vi "peg-in-hole 2015-03-12 Test.vi"() -> ()   [LabVIEW 2013]
uses:
  ROS/Code/SubVIs/BaxterSide.ctl
  Arm Globals.vi
  ROS/Code/Console/Servers/ServerSubs/(nist) Arm Globals.vi
panel:
  in  "Load Pick Pose":bool
  out "Pick Hole":T1={"X"=602.0, "Y"=-377.0, "Z"=10.0, "O"=0.0, "A"=0.0, "T"=0.0}
  in  "Pick Pose":dbl[](array[numeric])=[47.63671869556711, -52.91015618954133, -0.7470703116463477, 100.65673816623291, 0.6372070305218848, 42.143554639343975, 3.186035152609424]
  out "Loops Remaining":i32=1
  out "Peg":i32=1
  out "Times":dbl[](array[numeric])
  out "Status":string="Test.4"
  in  "Stop":bool
  out "error out":errorcluster
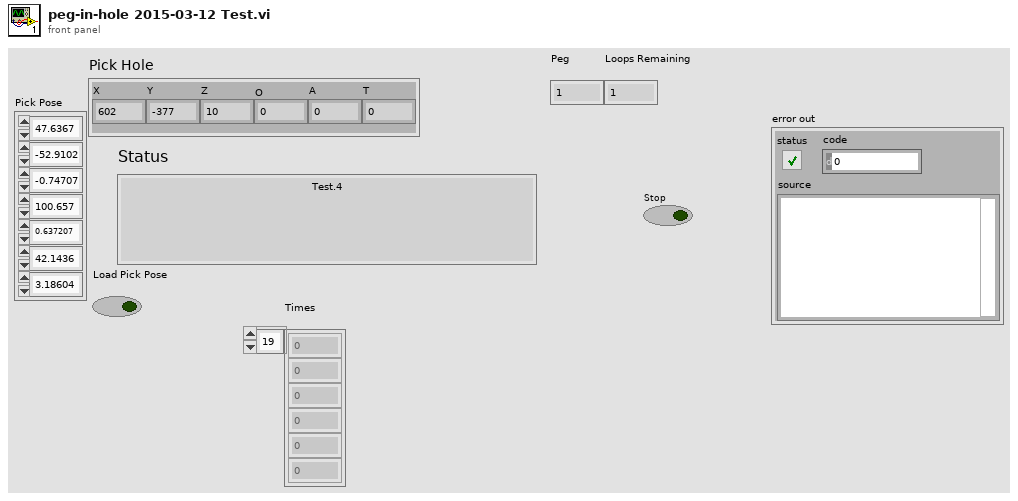
[diagram p1: front panel]
types:
  T1 = cluster{"X":dbl, "Y":dbl, "Z":dbl, "O":dbl, "A":dbl, "T":dbl}
  T2 = typedef "BaxterSide.ctl" = enum16{"left", "right"}
  T3 = cluster{"X":dbl, "Y":dbl, "Z":dbl, "O":dbl, "A":dbl, "T":dbl}[]
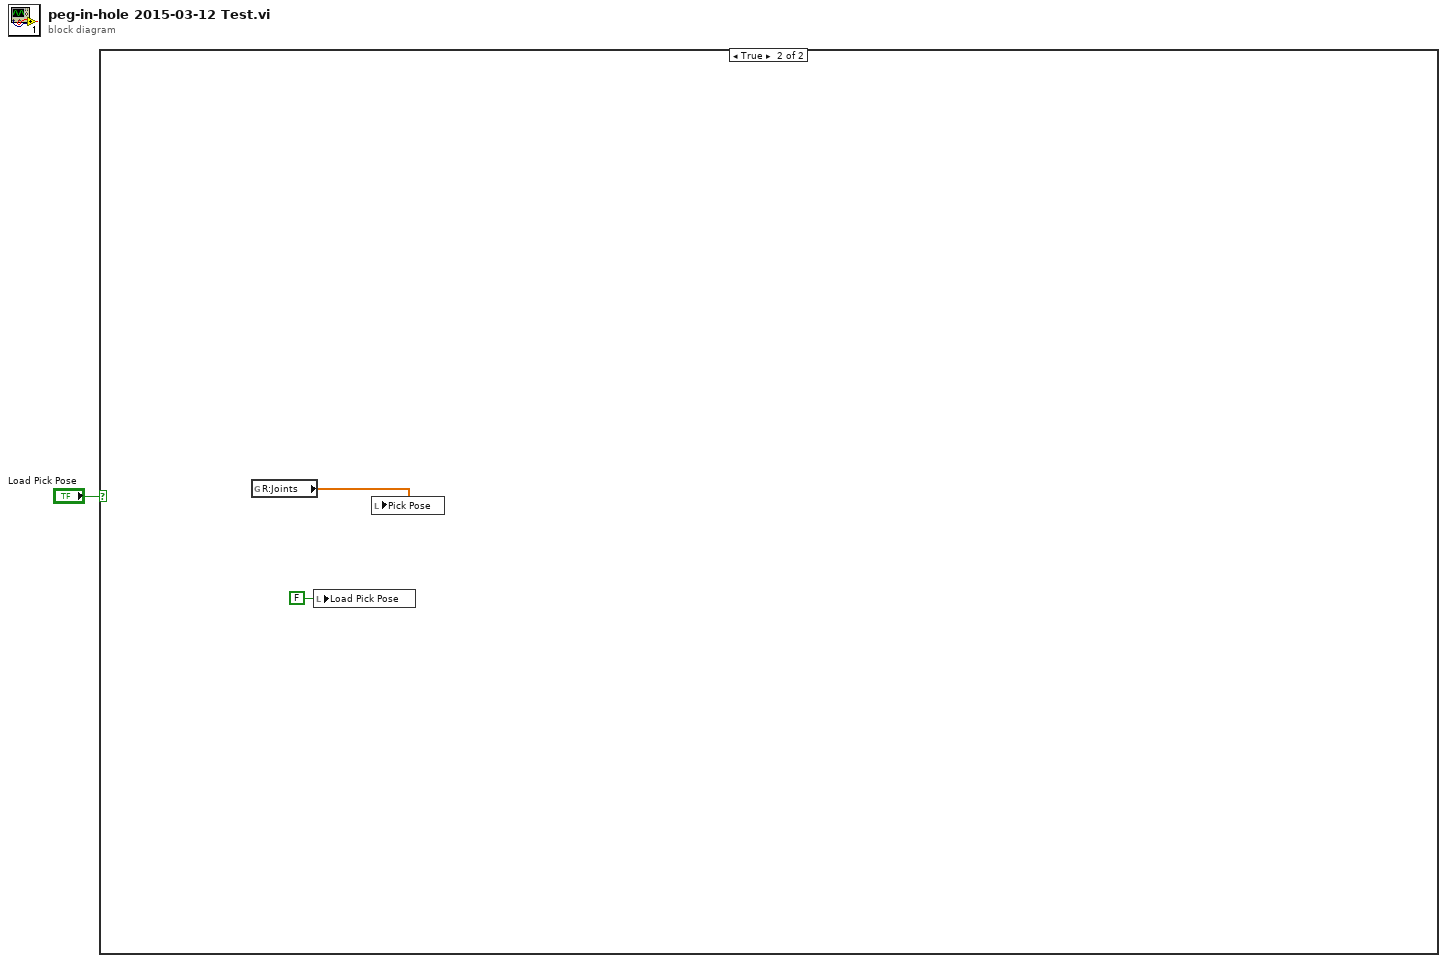
[diagram p0: block diagram]
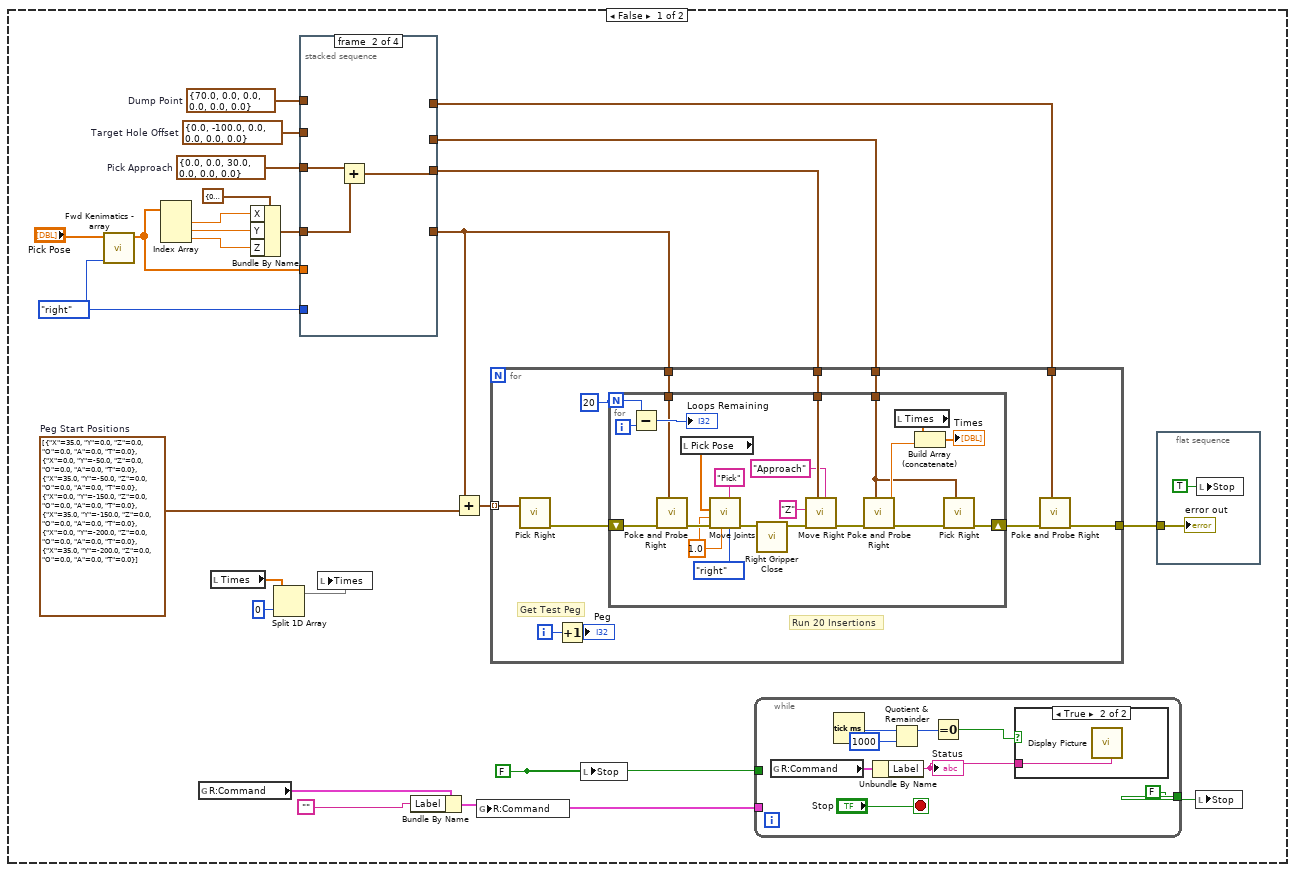
[diagram p2: hidden frame]
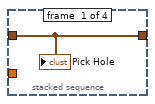
[diagram p3: hidden frame]
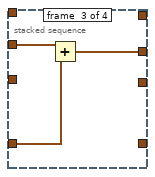
[diagram p4: hidden frame]
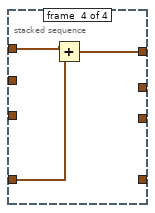
[diagram p5: hidden frame]
diagram:
  n1 = case shown="True" "Load Pick Pose" {
    frame False {
      w3 = T1 {"X"=0.0, "Y"=0.0, "Z"=30.0, "O"=0.0, "A"=0.0, "T"=0.0}  # Pick Approach
      w9 = T1 {"X"=70.0, "Y"=0.0, "Z"=0.0, "O"=0.0, "A"=0.0, "T"=0.0}  # Dump Point
      w10 = T1 {"X"=0.0, "Y"=-100.0, "Z"=0.0, "O"=0.0, "A"=0.0, "T"=0.0}  # Target Hole Offset
      w6 = BaxterSide."right" ("Side")
      w17 = T3 [{"X"=35.0, "Y"=0.0, "Z"=0.0, "O"=0.0, "A"=0.0, "T"=0.0}, {"X"=0.0, "Y"=-50.0, "Z"=0.0, "O"=0.0, "A"=0.0, "T"=0.0}, {"X"=35.0, "Y"=-50.0, "Z"=0.0, "O"=0.0, "A"=0.0, "T"=0.0}, {"X"=0.0, "Y"=-150.0, "Z"=0.0, "O"=0.0, "A"=0.0, "T"=0.0}, {"X"=35.0, "Y"=-150.0, "Z"=0.0, "O"=0.0, "A"=0.0, "T"=0.0}, {"X"=0.0, "Y"=-200.0, "Z"=0.0, "O"=0.0, "A"=0.0, "T"=0.0}, {"X"=35.0, "Y"=-200.0, "Z"=0.0, "O"=0.0, "A"=0.0, "T"=0.0}]  # Peg Start Positions
      w23 = FALSE ("Stop")
      n2 = call "Fwd Kenimatics - array.vi"("Side"=w6, "Joints"="Pick Pose") -> ("Position"=w7:dbl[])  [unwired: 8 in, 1 out]
      n3 = Index Array(array=w7) -> (element #1=w14:dbl, element #2=w13:dbl, element #3=w12:dbl)  [unwired: 3 in]
      n4 = global read "Arm Globals.vi" "R:Command"() -> (w27:cluster{"Label":string, "Angles":dbl[]})
      n5 = local read "Times"() -> (w21:dbl[])
      n6 = Bundle By Name(cluster=T1 {"X"=0.0, "Y"=0.0, "Z"=0.0, "O"=0.0, "A"=0.0, "T"=0.0} ("Pick Hole"), "X"=w14, "Y"=w13, "Z"=w12) -> (w11:T1)
      n7 = Split 1D Array(array=w21, index=0) -> (first subarray=w19:dbl[])  [unwired: 1 out]
      n8 = stacked-sequence {
        tunnel: w11 -> [w28 w30 w33 w36]
        tunnel: [w28 _ _ _] -> w5
        tunnel: w10 -> [_ _ w34 _]
        tunnel: [_ _ w32 _] -> w4
        tunnel: w9 -> [_ _ _ w37]
        tunnel: [_ _ _ w35] -> w8
        tunnel: w7 -> [_ _ _ _]
        tunnel: w6 -> [_ _ _ _]
        tunnel: w3 -> [_ w31 _ _]
        tunnel: [_ w29 _ _] -> w2
        frame #0 {
          "Pick Hole" <- w28
        }
        frame #1 {
          n9 = Add(x=w31, y=w30) -> (x+y=w29:T1)
        }
        frame #2 {
          n10 = Add(x=w34, y=w33) -> (x+y=w32:T1)
        }
        frame #3 {
          n11 = Add(x=w37, y=w36) -> (x+y=w35:T1)
        }
      }
      n12 = local write "Times"(w19) -> ()
      n13 = Bundle By Name(cluster=w27, "Label"="") -> (w25:cluster{"Label":string, "Angles":dbl[]})
      n14 = Add(x=w5, y=w17) -> (x+y=w18:T3)
      n15 = global write "Arm Globals.vi" "R:Command"(w25) -> ()
      n16 = for {
        tunnel: [w43] -> w22
        tunnel: w18 -> [w44] mode=indexing
        tunnel: w8 -> [w45]
        tunnel: w5 -> [w41]
        tunnel: w4 -> [w40]
        tunnel: w2 -> [w38]
        i -> [w46]
        # "Run 20 Insertions"
        # "Get Test Peg"
        n17 = call "Pick Right.vi"("Pick"=w44) -> ("error out"=w42:errorcluster)  [unwired: 10 in]
        n18 = Increment(x=w46) -> (x+1=→"Peg":i32)
        n19 = for {
          N: 20 -> [w68]
          shift-right: [w61] -> w39
          shift-left: w42 -> [w59]
          tunnel: w41 -> [w63]
          tunnel: w40 -> [w60]
          tunnel: w38 -> [w51]
          i -> [w67]
          w55 = 1.0 ("Wait (s)")
          n20 = Subtract(x=w68, y=w67) -> (x-y=→"Loops Remaining":i32)
          n21 = call "Poke and Probe Right.vi"("Start"=w63, "error in"=w59) -> ("error out"=w58:errorcluster)  [unwired: 8 in, 1 out]
          n22 = local read "Pick Pose"() -> (w56:dbl[])
          n23 = call "Move Joints.vi"("Side"=BaxterSide."right", "Label"="Pick", "Wait (s)"=w55, "error in"=w58, "time"=w55, "Goal"=w56) -> ("error out"=w54:errorcluster)  [unwired: 4 in, 1 out]
          n24 = call "Right Gripper Close.vi"("error in"=w54) -> ("error out"=w53:errorcluster)  [unwired: 9 in, 1 out]
          n25 = call "Move Right.vi"("Label"="Approach", "Goal Axes"=w51, "error in"=w53, "Mask"="Z") -> ("error out"=w52:errorcluster)  [unwired: 3 in, 4 out]
          n26 = call "Poke and Probe Right.vi"("Start"=w60, "error in"=w52) -> ("error out"=w62:errorcluster, "time"=w70:dbl)  [unwired: 8 in]
          n27 = local read "Times"() -> (w64:dbl[])
          n28 = Build Array (concatenate)(w64, w70) -> (→"Times":dbl[])
          n29 = call "Pick Right.vi"("Pick"=w60, "error in"=w62) -> ("error out"=w61:errorcluster)  [unwired: 9 in]
        }
        n30 = call "Poke and Probe Right.vi"("Start"=w45, "error in"=w39) -> ("error out"=w43:errorcluster)  [unwired: 8 in, 1 out]
      }
      n31 = local write "Stop"(w23) -> ()
      n32 = while {
        tunnel: w25 -> [_]
        tunnel: [FALSE] -> w24
        tunnel: w23 -> [_]
        stop <- "Stop" stop-if-true
        n33 = global read "Arm Globals.vi" "R:Command"() -> (w80:cluster{"Label":string, "Angles":dbl[]})
        n34 = Tick Count (ms)() -> (millisecond timer value=w77:u32)
        n35 = Unbundle By Name(w80) -> ("Label"=w73:string)
        "Status" <- w73
        n36 = Quotient & Remainder(x=w77, y=u32 1000) -> (x-y*floor(x/y)=w75:u32)  [unwired: 1 out]
        n37 = Equal To 0?(x=w75) -> (x = 0?=w74:bool)
        n38 = case shown="True" w74 {
          tunnel: w73 -> [_ w81]
          frame False {
          }
          frame True {
            n39 = call "Display Picture.vi"("Comment"=w81) -> ()  [unwired: 10 in, 1 out]
          }
        }
      }
      n40 = flat-sequence {
        tunnel: w22 -> [w72]
        frame #0 {
          n41 = local write "Stop"(TRUE ("Stop")) -> ()
          "error out" <- w72
        }
      }
      n42 = local write "Stop"(w24) -> ()
    }
    frame True {
      n43 = global read "(nist) Arm Globals.vi" "R:Joints"() -> (w83:dbl[])
      n44 = local write "Load Pick Pose"(FALSE ("Load Pick Pose")) -> ()
      n45 = local write "Pick Pose"(w83) -> ()
    }
  }
